vi "Plot GetEmbeddedString.vi"(11 "Start String":string) -> (1 "Error":bool, 2 "EmbeddedString":string, 3 "Remaining String":string)   [LabVIEW 2020, in "3D Plot.lvclass"]
uses:
  3D Plot.lvclass
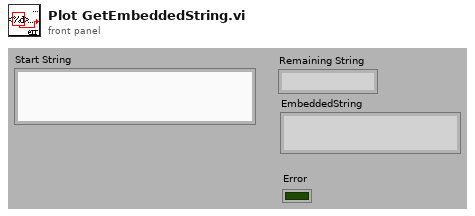
[diagram p1: front panel]
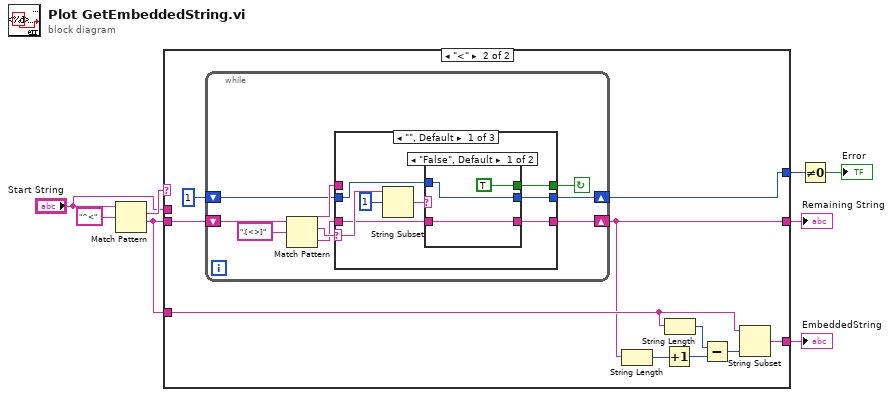
[diagram p0: block diagram]
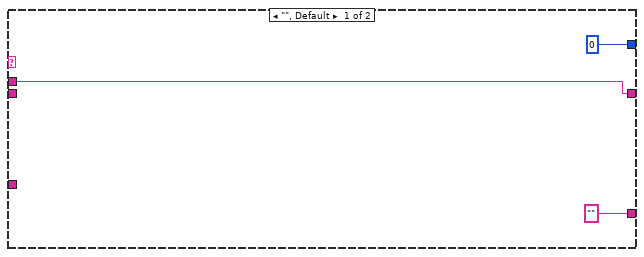
[diagram p2: hidden frame]
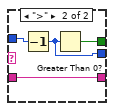
[diagram p3: hidden frame]
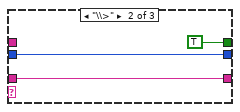
[diagram p4: hidden frame]
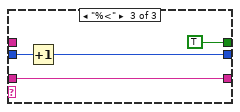
[diagram p5: hidden frame]
diagram:
  n1 = Match Pattern(string="Start String", regular expression="^<") -> (match substring=w7:string, after substring=w4:string)  [unwired: 3 out]
  n2 = case shown="\"<\"" w7 {
    tunnel: w4 -> [_ w20]
    tunnel: [w11 w16] -> w6
    tunnel: "Start String" -> [w11 _]
    tunnel: [0 w19] -> w2
    tunnel: w4 -> [_ w18]
    tunnel: ["" ("Start String") w17] -> w3
    frame "", Default {
    }
    frame "<" {
      n3 = while {
        shift-right: [w25] -> w19
        shift-left: 1 -> [w26]
        shift-right: [w22] -> w16
        shift-left: w20 -> [w30]
        stop <- w24 continue-if-true
        n4 = Match Pattern(string=w30, regular expression=".[<>]") -> (before substring=w27:string, match substring=w28:string, after substring=w23:string)  [unwired: 2 out]
        n5 = case shown="\"\", Default" w28 {
          selector: w28 -> [w37 _ _]
          tunnel: w27 -> [_ _ _]
          tunnel: w26 -> [w34 w46 w52]
          tunnel: [w33 w46 w51] -> w25
          tunnel: [w38 TRUE TRUE] -> w24
          tunnel: w23 -> [w31 w48 w49]
          tunnel: [w32 w48 w49] -> w22
          frame "", Default {
            n6 = String Subset(string=w37, offset (0)=1) -> (substring=w35:string)  [unwired: 1 out]
            n7 = case shown="\"False\", Default" w35 {
              tunnel: [TRUE w43] -> w38
              tunnel: w34 -> [w41 w45]
              tunnel: [w41 w44] -> w33
              tunnel: [w40 w42] -> w32
              tunnel: w31 -> [w40 w42]
              frame "False", Default {
              }
              frame ">" {
                n8 = Decrement(x=w45) -> (x-1=w44:i32)
                n9 = Greater Than 0?(x=w44) -> (x > 0?=w43:bool)
              }
            }
          }
          frame "\\>" {
          }
          frame "%<" {
            n10 = Increment(x=w52) -> (x+1=w51:i32)
          }
        }
      }
      n11 = String Length(string=w16) -> (length=w15:i32)
      n12 = Increment(x=w15) -> (x+1=w13:i32)
      n13 = String Length(string=w18) -> (length=w14:i32)
      n14 = Subtract(x=w14, y=w13) -> (x-y=w12:i32)
      n15 = String Subset(string=w18, length (rest)=w12) -> (substring=w17:string)  [unwired: 1 out]
    }
  }
  "Remaining String" <- w6
  "EmbeddedString" <- w3
  n16 = Not Equal To 0?(x=w2) -> (x != 0?=→"Error":bool)
